vi "Cooling.vi"(6 "Read Field":bool, 7 "Read Fan":bool, 8 "Field":T1, 9 "Cluster":T3={"Set point (*C)"=0, "Sample temperature (*C)"=0, "Datafile blob"="8/29/2014\t3:28 PM\r\n\r\n0*C\r\nH2-CO2\r\nIW/IM+0\r\n\r\nTime\tSet_point\tLoad_end\tSample\tFan_end\tFan\tField\t%CO2\r\n", "Email address"="", "refnum out"=refnum, "Email"=FALSE}, 11 "Ports":T2={"Oven Watlows"="COM1", "Field Power Supply"="COM9", "Oven Fan"="COM4", "Flow Controllers"="COM3"}) -> (0 "Fan on":bool, 1 "stop":bool, 3 "Field on":bool, 4 "Cool":bool, 5 "Current SP":dbl=50.0)   [LabVIEW 2009]
panel:
  out "Run complete":bool
  # "Input"
  # "Output"
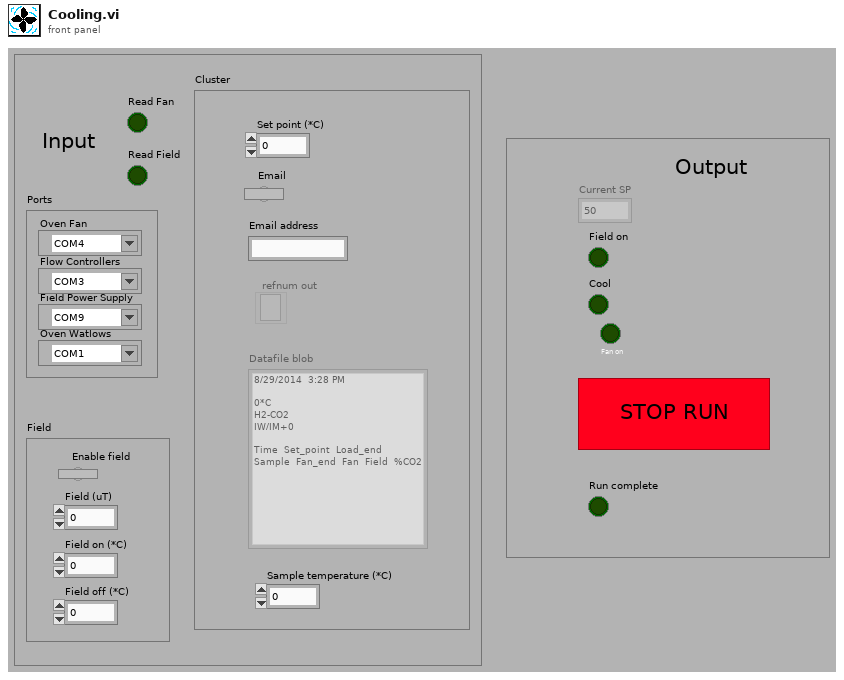
[diagram p1: front panel]
types:
  T1 = cluster{"Field on (*C)":dbl, "Field off (*C)":dbl, "Field (uT)":dbl, "Enable field":bool}
  T2 = cluster{"Oven Watlows":refnum<visa-resource-name>, "Field Power Supply":refnum<visa-resource-name>, "Oven Fan":refnum<visa-resource-name>, "Flow Controllers":refnum<visa-resource-name>}
  T3 = cluster{"Set point (*C)":u32, "Sample temperature (*C)":u32, "Datafile blob":string, "Email address":string, "refnum out":refnum<file>, "Email":bool}
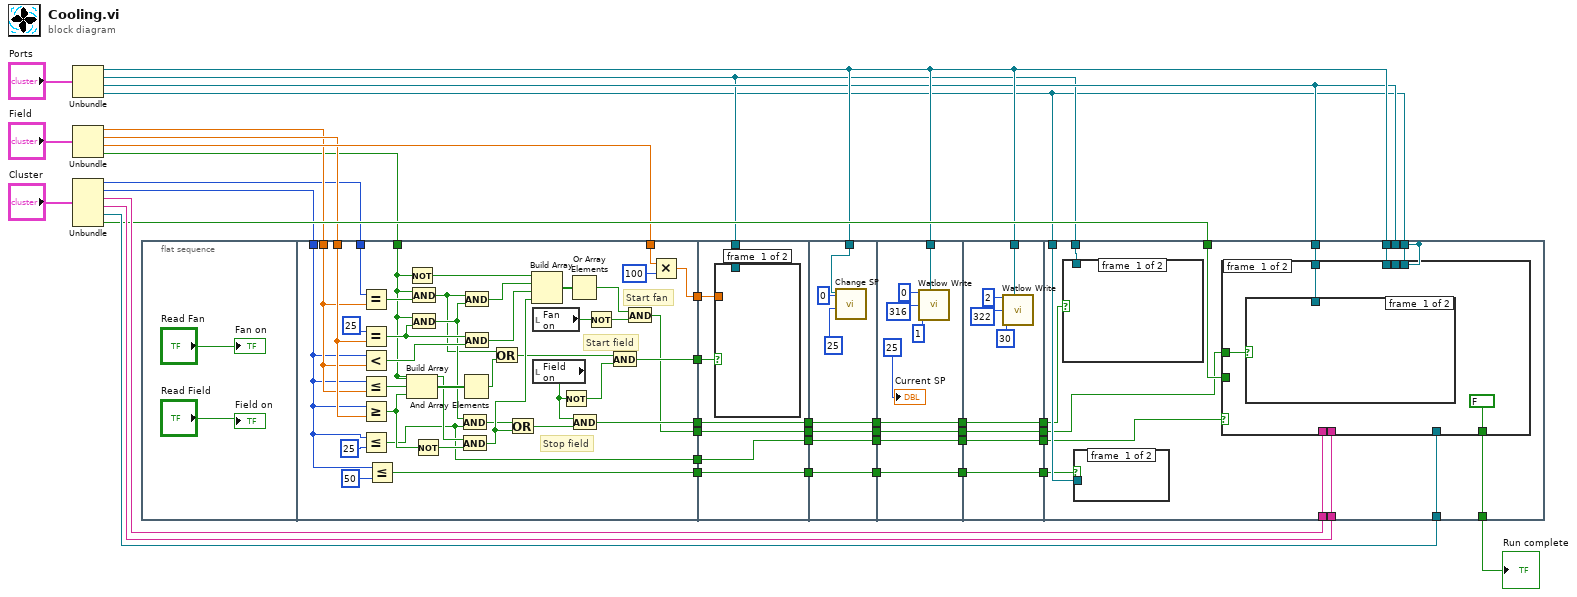
[diagram p0: block diagram]
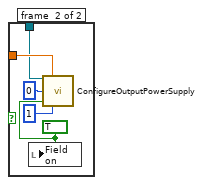
[diagram p2: hidden frame]
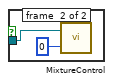
[diagram p3: hidden frame]
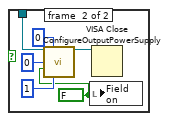
[diagram p4: hidden frame]
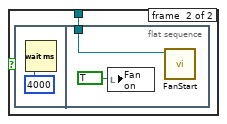
[diagram p5: hidden frame]
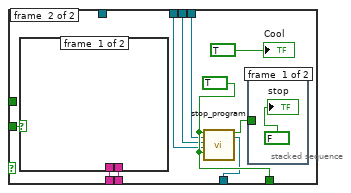
[diagram p6: hidden frame]
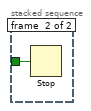
[diagram p7: hidden frame]
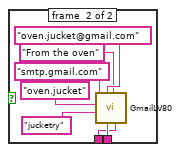
[diagram p8: hidden frame]
diagram:
  n1 = Unbundle("Ports") -> ("Oven Watlows"=w4:refnum<visa-resource-name>, "Field Power Supply"=w2:refnum<visa-resource-name>, "Oven Fan"=w3:refnum<visa-resource-name>, "Flow Controllers"=w1:refnum<visa-resource-name>)
  n2 = Unbundle("Field") -> ("Field on (*C)"=w28:dbl, "Field off (*C)"=w29:dbl, "Field (uT)"=w30:dbl, "Enable field"=w26:bool)
  n3 = Unbundle("Cluster") -> ("Set point (*C)"=w27:u32, "Sample temperature (*C)"=w25:u32, "Datafile blob"=w34:string, "Email address"=w35:string, "refnum out"=w36:refnum<file>, "Email"=w33:bool)
  n4 = flat-sequence {
    tunnel: [w56] -> w32
    tunnel: [w55] -> w31
    tunnel: w30 -> [w54]
    tunnel: w29 -> [w53]
    tunnel: w28 -> [w52]
    tunnel: w27 -> [w51]
    tunnel: w26 -> [w50]
    tunnel: w25 -> [w49]
    tunnel: [w46] -> w20
    tunnel: [w45] -> w15
    tunnel: [w44] -> w10
    tunnel: [w43] -> w9
    tunnel: w2 -> [w88]
    tunnel: w32 -> [w87]
    tunnel: w31 -> [w86]
    tunnel: [w85] -> w21
    tunnel: w20 -> [w85]
    tunnel: [w84] -> w16
    tunnel: w15 -> [w84]
    tunnel: [w83] -> w11
    tunnel: w10 -> [w83]
    tunnel: w9 -> [w82]
    tunnel: [w82] -> w8
    tunnel: w4 -> [w94]
    tunnel: [w98] -> w22
    tunnel: w21 -> [w98]
    tunnel: [w97] -> w17
    tunnel: w16 -> [w97]
    tunnel: [w96] -> w12
    tunnel: w11 -> [w96]
    tunnel: w8 -> [w95]
    tunnel: [w95] -> w7
    tunnel: w4 -> [w106]
    tunnel: [w104] -> w23
    tunnel: w22 -> [w104]
    tunnel: [w103] -> w18
    tunnel: w17 -> [w103]
    tunnel: [w102] -> w13
    tunnel: w12 -> [w102]
    tunnel: w7 -> [w101]
    tunnel: [w101] -> w6
    tunnel: w4 -> [w114]
    tunnel: [w113] -> w24
    tunnel: w23 -> [w113]
    tunnel: [w112] -> w19
    tunnel: w18 -> [w112]
    tunnel: [w111] -> w14
    tunnel: w13 -> [w111]
    tunnel: w6 -> [w110]
    tunnel: [w110] -> w5
    tunnel: w36 -> [w132]
    tunnel: [w131] -> w40
    tunnel: w2 -> [w130]
    tunnel: [w118] -> _
    tunnel: w4 -> [w129]
    tunnel: w3 -> [w128]
    tunnel: w1 -> [w127]
    tunnel: w33 -> [w126]
    tunnel: w1 -> [w125]
    tunnel: w35 -> [w124]
    tunnel: w34 -> [w123]
    tunnel: w24 -> [w122]
    tunnel: w19 -> [w121]
    tunnel: w14 -> [w120]
    tunnel: w5 -> [w119]
    tunnel: w3 -> [w118]
    frame #0 {
      "Fan on" <- "Read Fan"
      "Field on" <- "Read Field"
    }
    frame #1 {
      # "Stop field"
      # "Start field"
      # "Start fan"
      n5 = Equal?(x=w51, y=w52) -> (x = y?=w59:bool)
      n6 = Equal?(x=25, y=w53) -> (x = y?=w74:bool)
      n7 = Less?(x=w49, y=w52) -> (x < y?=w75:bool)
      n8 = Less Or Equal?(x=w49, y=w52) -> (x <= y?=w79:bool)
      n9 = Greater Or Equal?(x=w49, y=w53) -> (x >= y?=w78:bool)
      n10 = Less Or Equal?(x=w49, y=25) -> (x <= y?=w44:bool)
      n11 = Less Or Equal?(x=w49, y=50) -> (x <= y?=w45:bool)
      n12 = Not(x=w50) -> (.not. x?=w71:bool)
      n13 = Build Array(w50, w79, w78) -> (w77:bool[])
      n14 = And(x=w50, y=w59) -> (x .and. y?=w60:bool)
      n15 = And(x=w50, y=w74) -> (x .and. y?=w64:bool)
      n16 = Not(x=w78) -> (.not. x?=w61:bool)
      n17 = And(x=w64, y=w44) -> (x .and. y?=w65:bool)
      n18 = And(x=w50, y=w61) -> (x .and. y?=w81:bool)
      n19 = And Array Elements(Boolean array=w77) -> (logical AND=w80:bool)
      n20 = And(x=w60, y=w64) -> (x .and. y?=w72:bool)
      n21 = And(x=w74, y=w75) -> (x .and. y?=w70:bool)
      n22 = Or(x=w60, y=w80) -> (x .or. y?=w62:bool)
      n23 = Or(x=w65, y=w81) -> (x .or. y?=w76:bool)
      n24 = Build Array(w71, w72, w70, w81) -> (w68:bool[])
      n25 = local read "Fan on"() -> (w48:bool)
      n26 = local read "Field on"() -> (w47:bool)
      n27 = Not(x=w47) -> (.not. x?=w63:bool)
      n28 = Or Array Elements(Boolean array=w68) -> (logical OR=w69:bool)
      n29 = And(x=w47, y=w76) -> (x .and. y?=w46:bool)
      n30 = Not(x=w48) -> (.not. x?=w66:bool)
      n31 = And(x=w62, y=w63) -> (x .and. y?=w55:bool)
      n32 = And(x=w69, y=w66) -> (x .and. y?=w43:bool)
      n33 = Multiply(x=w54, y=100) -> (x*y=w56:dbl)
    }
    frame #2 {
      n34 = case shown="True" w86 {
        tunnel: w87 -> [_ w91]
        tunnel: w88 -> [_ w90]
        frame #0 {
        }
        frame #1 {
          w89 = TRUE
          n35 = local write "Field on"(w89) -> ()
          n36 = call "ConfigureOutputPowerSupply.vi"("VISA resource name"=w90, "Manual Range(0.00)"=w91, "Function(0:Voltage)"=0, "Output Enable (T: Enable)"=w89, "Unit(V)"=1) -> ()  [unwired: 9 in, 2 out]
        }
      }
    }
    frame #3 {
      n37 = call "Change SP.vi"("Set Point"=25, "Adress"=0, "VISA resource name"=w94) -> ()  [unwired: 1 in, 1 out]
    }
    frame #4 {
      n38 = call "Watlow Write.vi"("Adress"=0, "VISA resource name"=w106, "Register"=u16 316 ("ST-H"), "Parameter"=1) -> ()  [unwired: 1 in, 1 out]
      "Current SP" <- 25
    }
    frame #5 {
      n39 = call "Watlow Write.vi"("Adress"=2, "VISA resource name"=w114, "Register"=u16 322 ("ST-H"), "Parameter"=30) -> ()  [unwired: 1 in, 1 out]
    }
    frame #6 {
      n40 = case shown="False" w122 {
        tunnel: w130 -> [_ w136]
        frame #0 {
        }
        frame #1 {
          w135 = FALSE
          n41 = call "ConfigureOutputPowerSupply.vi"("VISA resource name"=w136, "Manual Range(0.00)"=0, "Function(0:Voltage)"=0, "Output Enable (T: Enable)"=w135, "Unit(V)"=1) -> ("VISA resource name out"=w140:refnum<visa-resource-name>)  [unwired: 9 in, 1 out]
          n42 = local write "Field on"(w135) -> ()
          n43 = VISA Close(VISA resource name=w140) -> ()  [unwired: 1 in, 1 out]
        }
      }
      n44 = case shown="True" w121 {
        tunnel: w127 -> [_ w133]
        frame #0 {
        }
        frame #1 {
          n45 = call "MixtureControl.vi"("%CO2"=0, "VISA resource name"=w133) -> ()  [unwired: 1 in]
        }
      }
      n46 = case shown="True" w120 {
        tunnel: w132 -> [_ w152]
        tunnel: w119 -> [w143 _]
        tunnel: [FALSE w156] -> w131
        tunnel: w118 -> [_ w155]
        tunnel: w129 -> [_ w154]
        tunnel: w128 -> [w141 _]
        tunnel: w126 -> [_ w148]
        tunnel: w125 -> [_ w151]
        tunnel: w124 -> [_ w150]
        tunnel: w123 -> [_ w149]
        frame #0 {
          n47 = case shown="True" w143 {
            tunnel: w141 -> [_ w144]
            frame #0 {
            }
            frame #1 {
              n48 = flat-sequence {
                tunnel: w144 -> [w146]
                frame #0 {
                  n49 = Wait (ms)(milliseconds to wait=4000) -> ()  [unwired: 1 out]
                }
                frame #1 {
                  n50 = local write "Fan on"(TRUE) -> ()
                  n51 = call "FanStart.vi"("VISA resource name"=w146) -> ()  [unwired: 11 in]
                }
              }
            }
          }
        }
        frame #1 {
          w156 = TRUE
          n52 = case shown="True" w148 {
            tunnel: w150 -> [_ w161]
            tunnel: w149 -> [_ w160]
            frame #0 {
            }
            frame #1 {
              n53 = call "GmailLV80.vi"("Body"=w160, "Subject"="From the oven", "Recipient's Email Address"=w161, "Sender's Email Address (eg: LabVIEW@gmail.com)"="oven.jucket@gmail.com", "GMAIL Account Password"="jucketry", "GMAIL Account User ID"="oven.jucket", "Outgoing Mail Server (SMTP)"="smtp.gmail.com") -> ()  [unwired: 1 in, 4 out]
            }
          }
          n54 = call "stop_program.vi"("Run complete"=w156, "Flow Controllers"=w151, "Fan"=w155, "Watlows"=w154, "stop"=w156, "filename"=w152) -> ("Reset?"=w157:bool)  [unwired: 12 in, 1 out]
          n55 = stacked-sequence {
            tunnel: w157 -> [_ w159]
            frame #0 {
              "stop" <- FALSE
            }
            frame #1 {
              n56 = Stop(stop? (T)=w159) -> ()
            }
          }
          "Cool" <- TRUE
        }
      }
    }
  }
  "Run complete" <- w40
